vi "Write control param.vi"(8 "error in (no error)":errorcluster, 10 "control param":T1={"proportional gain (Kc)"=1.0, "integral time (Ti, s)"=10.0, "derivative time (Td, s)"=1.0, "output high"=100.0, "output high start"=40.0, "output high stop"=40.0, "alr value"=0.0, "output low"=0.0, "output rate (EGU/s)"=5.0, "setpoint max"=100.0, "setpoint rate (EGU/min)"=10.0, "stop rate (EGU/min)"=5.0} {"setpoint max" format="%.2f"; "stop rate (EGU/min)" min=0.001 format="%.2f"; "setpoint rate (EGU/min)" min=0.001 format="%.2f"; "output high stop" format="%.2f"; "output high start" format="%.2f"; "output rate (EGU/s)" min=0.001 format="%.2f"; "output low" format="%.2f"; "alr value" format="%.2f"; "output high" format="%.2f"; "derivative time (Td, s)" format="%.3f"; "integral time (Ti, s)" format="%.3f"; "proportional gain (Kc)" format="%.3f"}, 11 "reg in":refnum<class "bronkhorst_reg.lvclass">) -> (0 "error out":errorcluster, 3 "reg out":refnum<class "bronkhorst_reg.lvclass">)   [LabVIEW 2019, in "bronkhorst_reg.lvclass"]
uses:
  bronkhorst_reg.lvclass
  ctl/control param.ctl
  bronkhorst_reg.lvclass/bronkhorst_reg.ctl
  control.lvlib
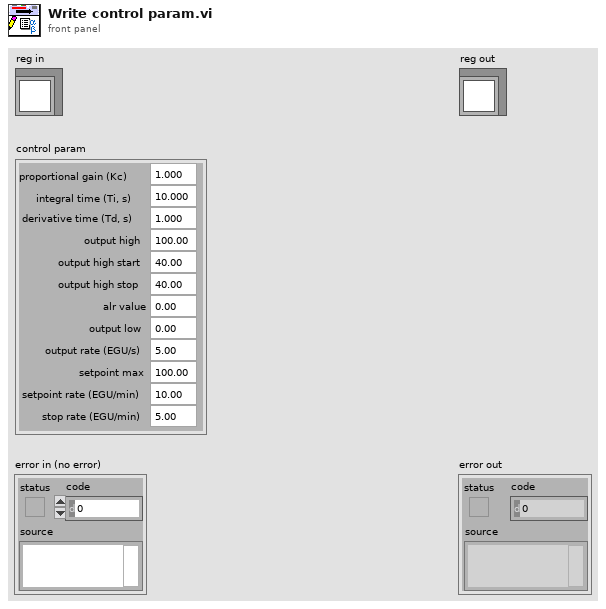
[diagram p1: front panel]
types:
  T1 = typedef "control.lvlib/control param.ctl" = cluster{"proportional gain (Kc)":dbl, "integral time (Ti, s)":dbl, "derivative time (Td, s)":dbl, "output high":dbl, "output high start":dbl, "output high stop":dbl, "alr value":dbl, "output low":dbl, "output rate (EGU/s)":dbl, "setpoint max":dbl, "setpoint rate (EGU/min)":dbl, "stop rate (EGU/min)":dbl}
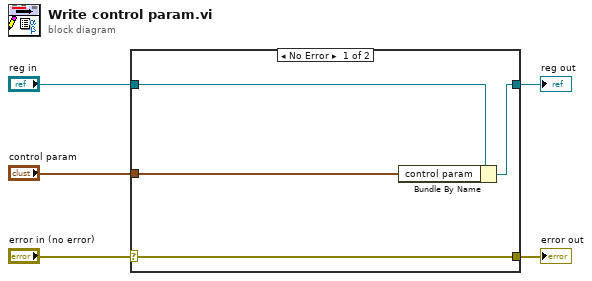
[diagram p0: block diagram]
diagram:
  n1 = case shown="No Error" "error in (no error)" {
    selector: "error in (no error)" -> [w9 w10]
    tunnel: [w9 w10] -> w4
    tunnel: [w7 w11] -> w2
    tunnel: "reg in" -> [w8 w11]
    tunnel: "control param" -> [w6 _]
    frame No Error {
      n2 = Bundle By Name(cluster=w8, "control param"=w6) -> (w7:refnum<class "bronkhorst_reg.lvclass">)
    }
    frame Error {
    }
  }
  "error out" <- w4
  "reg out" <- w2
